vi "test_ThreeSessThreePinTwoInstrTwoSiteReservation_CallGetConnectionsFromPinsForOneFgenPinAllSites_ReturnsOneConnection.vi"(8 "error in":errorcluster) -> (0 "error out":errorcluster, 2 "result":string, 3 "pass":bool)   [LabVIEW 2020, in "MeasurementServerTests.lvlib"]
uses:
  MeasurementServerTests.lvlib
  Runtime/Clients/Session Management V1/Session Reservation/Connection.ctl
  Runtime/Clients/Session Management V1/Session Reservation/Session Reservation.lvclass
  Runtime/Clients/Session Management V1/Session Reservation/Connection with Session.ctl
  c3cb69a0-23cd-49fc-99d1-8c54773f0200.vi
  7916252b-9f70-410a-a363-a2f79f13546d.vi
  Runtime/Sessions/niFGEN Sessions/Session Factory/Session Factory.lvclass
  Runtime/Clients/Session Management V1/Session Reservation/Pin Type.ctl
  1892c976-b1e4-4620-b87e-3b80d3940375.vi
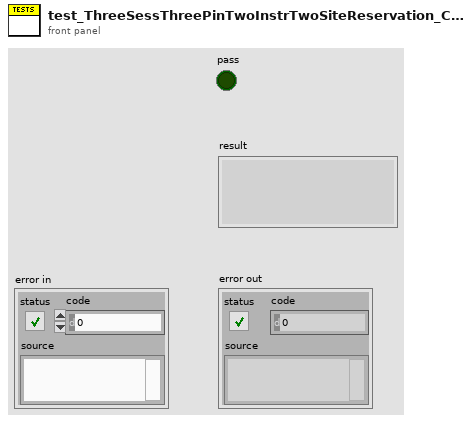
[diagram p1: front panel]
types:
  T1 = typedef "NI Session Management V1 Client.lvlib/Session Reservation.lvclass/Pin Type.ctl" = enum16{"DUT and System Pins", "System Pins"}
  T2 = typedef "NI Session Management V1 Client.lvlib/Session Reservation.lvclass/Connection.ctl" = cluster{"pin or relay name":string, "site":i32, "instrument type id":string, "channel":string}
  T3 = typedef "NI Session Management V1 Client.lvlib/Session Reservation.lvclass/Connection with Session.ctl" = cluster{"connection":T2, "session":variant}
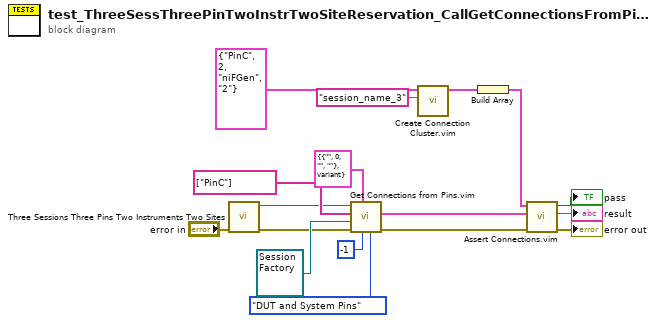
[diagram p0: block diagram]
diagram:
  n1 = call "Three Sessions Three Pins Two Instruments Two Sites.vi"("error in"="error in") -> ("error out"=w4:errorcluster, "session reservation out"=w3:refnum<class "Session Reservation.lvclass">)  [unwired: 8 in, 1 out]
  n2 = call "Get Connections from Pins.vim"("pin type"=Pin_Type."DUT and System Pins", "site"=-1, "connection type"=T3 {"connection"={"pin or relay name"="", "site"=0, "instrument type id"="", "channel"=""}, "session"=variant} ("connection"), "error in"=w4, "session factory"=refnum<class "Session Factory.lvclass"> refnum ("MeasurementLink niFGEN.lvlib:Instrument.lvclass"), "pin or relay names"=string[] ["PinC"], "session reservation in"=w3) -> ("error out"=w2:errorcluster, "connections"=w15:T3[])  [unwired: 2 in, 1 out]
  n3 = call "Create Connection Cluster.vim"("session in"="session_name_3", "hardware independent connection in"=T2 {"pin or relay name"="PinC", "site"=2, "instrument type id"="niFGen", "channel"="2"} ("connection")) -> ("connection out"=w11:T3)  [unwired: 9 in]
  n4 = Build Array(w11) -> (w10:T3[])
  n5 = call "Assert Connections.vim"("error in"=w2, "actual connections"=w15, "expected connections"=w10) -> ("error out"=→"error out":errorcluster, "result"=→"result":string, "pass"=→"pass":bool)  [unwired: 6 in]
